vi "Test Create UA Server Tree.vi"(8 "Error In":errorcluster, 11 "Server Connection Information":T1) -> (0 "Error Out":errorcluster)   [LabVIEW 2017, in "Unit Tests.lvlib"]
uses:
  Unit Tests.lvlib
  source/Browser Core/Server Classes/UA Server/Server Connection Information.ctl
  source/Browser Core/Server Classes/UA Server/UA Server.lvclass/UA Server.ctl
  source/Browser Core/Server Classes/UA Server/UA Server.lvclass
  C:/Users/MattJ/Desktop/GitHubSCM/UA-Server-Browser/source/Browser Core/Server Classes/Base Tree/Base Tree.lvclass
  <vilib>/addons/_JKI Toolkits/Caraya/classes/Test/Test.lvclass
  <vilib>/addons/_JKI Toolkits/Caraya/classes/Assert/Assert.lvclass
  source/Browser Core/Server Classes/Base Tree/Base Tree.lvclass
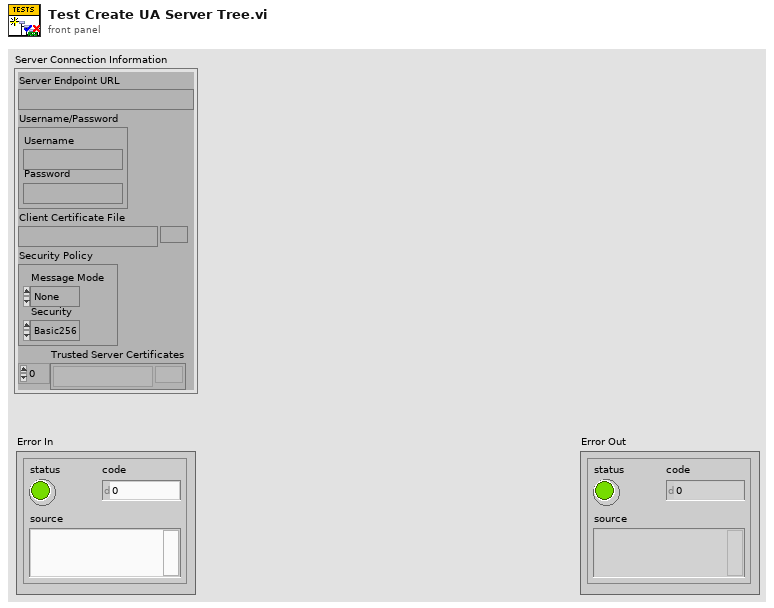
[diagram p1: front panel]
types:
  T1 = typedef "Browser Core.lvlib/UA Server.lvclass/Server Connection Information.ctl" = cluster{"Server Endpoint URL":string, "Username/Password":cluster{"Username":string, "Password":string}, "Client Certificate File":path, "Security Policy":cluster{"Message Mode":enum16{"None", "Sign", "Sign and Encrypt"}, "Security":enum16{"Basic256", "Basic128Rsa15"}}, "Trusted Server Certificates":path[]}
  T2 = cluster{"Message Mode":enum16{"None", "Sign", "Sign and Encrypt"}, "Security":enum16{"Basic256", "Basic128Rsa15"}}
  T3 = typedef "OPC UA Client Refnum.ctl" = refnum<k21>
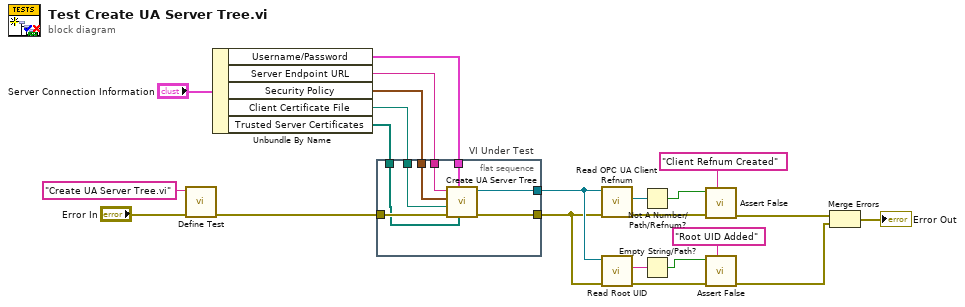
[diagram p0: block diagram]
diagram:
  n1 = call <vilib>:"Define Test.vi"("error in (no error)"="Error In", "Label (VI Title)"="Create UA Server Tree.vi") -> ("error out"=w20:errorcluster)  [unwired: 9 in]
  n2 = Unbundle By Name("Server Connection Information") -> ("Username/Password"=w1:cluster{"Username":string, "Password":string}, "Server Endpoint URL"=w18:string, "Security Policy"=w17:T2, "Client Certificate File"=w16:path, "Trusted Server Certificates"=w2:path[])
  n3 = flat-sequence "VI Under Test" {
    tunnel: w20 -> [w30]
    tunnel: w18 -> [w29]
    tunnel: w17 -> [w25]
    tunnel: w16 -> [w24]
    tunnel: [w28] -> w9
    tunnel: [w27] -> w10
    tunnel: w2 -> [w23]
    tunnel: w1 -> [w26]
    frame #0 {
      n4 = call "Create UA Server Tree.vi"("Trusted Server Certificates"=w23, "Username/Password"=w26, "Error In"=w30, "Client Certificate File"=w24, "Security Policy"=w25, "Server Endpoint URL"=w29) -> ("Error Out"=w28:errorcluster, "UA Server Tree"=w27:refnum<class "UA Server.lvclass">)  [unwired: 4 in]
    }
  }
  n5 = call "Read OPC UA Client Refnum.vi"("error in (no error)"=w9, "UA Server in"=w10) -> ("error out"=w15:errorcluster, "OPC UA client refnum"=w13:T3)  [unwired: 7 in, 1 out]
  n6 = call "Read Root UID.vi"("error in (no error)"=w9, "Base Tree in"=w10) -> ("error out"=w7:errorcluster, "Root UID"=w8:string)  [unwired: 7 in, 1 out]
  n7 = Not A Number/Path/Refnum?(number/path/refnum=w13) -> (NaN/Path/Refnum?=w12:bool)
  n8 = Empty String/Path?(string/path=w8) -> (empty?=w6:bool)
  n9 = call <vilib>:"Assert False.vi"("Label"="Client Refnum Created", "error in (no error)"=w15, "False?"=w12) -> ("error out"=w14:errorcluster)  [unwired: 8 in]
  n10 = call <vilib>:"Assert False.vi"("Label"="Root UID Added", "error in (no error)"=w7, "False?"=w6) -> ("error out"=w3:errorcluster)  [unwired: 8 in]
  n11 = Merge Errors(w14, w3) -> (→"Error Out":errorcluster)
